vi "PCO_GetImageEx.vi"(8 "error in (no error)":errorcluster, 10 "sBufNr":i16, 11 "Handle":u64) -> (0 "error out":errorcluster, 3 "Handle Out":u64, 5 "return type":u32 format="%x")   [LabVIEW 2011]
uses:
  SC2_Cam64.dll
panel:
  in  "Segment":u16
  in  "BitPerPixel":u16=14
  in  "YRes":u16=1040
  in  "XRes":u16=1368
  in  "LastImage":u32
  in  "1stImage":u32
  # "• wSegment: set to a segment number 1,2,3 or 4\n• dw1stImage (1 based index: 1…max available):\n• x = has to be a valid image number. If you try to access image e.g. 1 set this value to 1. (see \nPCO_GetNumberOfImagesInSegment).\n• dwLastImage (1 based index: dw1stImage…max available):\n• x = has to be a valid image number. If you try to access image e.g. 1 set this value to 1. (see \nPCO_GetNumberOfImagesInSegment).\n• sBufNr:\n• 0 … 7:.number of desired buffer.\n• wXRes: Actual x-Resolution of the image which should be transferred.\n• wYRes: Actual y-Resolution of the image which should be transferred.\n•WBitPerPixel: BitResolution of the image which should be transferred"
  # "will return for sure after 5s (with timeout)"
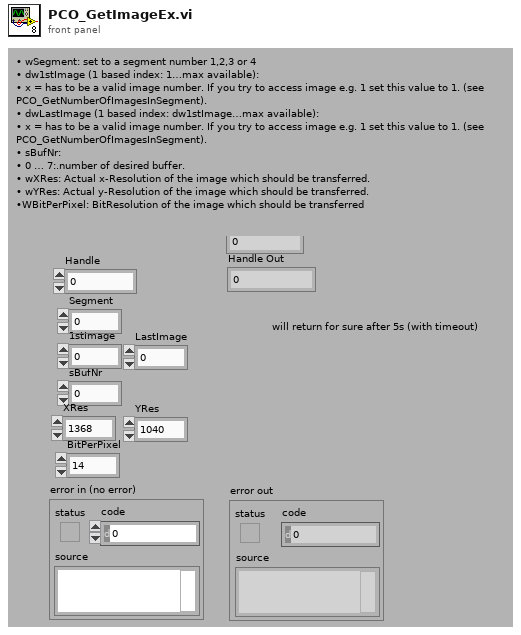
[diagram p1: front panel]
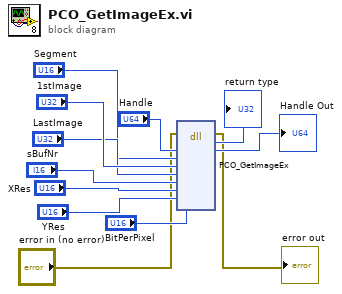
[diagram p0: block diagram]
diagram:
  n1 = dll-call lib="SC2_Cam*.*" fn="PCO_GetImageEx"(error in="error in (no error)", "Handle"="Handle", "Segment"="Segment", "1stImage"="1stImage", "LastImage"="LastImage", "sBufNr"="sBufNr", "XRes"="XRes", "YRes"="YRes", "BitPerPixel"="BitPerPixel") -> (error out=→"error out":errorcluster, "return type"=→"return type":u32, "Handle"=→"Handle Out":u64)  [unwired: 9 in, 1 out]
